vi "故障告警分析.vi"(8 "告警代码":u16, 9 "故障代码":u16, 10 "运行步序":u16, 11 "参数":string) -> (2 "报警内容":T1, 3 "简易报警状态":cluster{"故障状态":string, "报警状态":string}, 5 "platform_alarm_code":string)   [LabVIEW 2016, in "斯坦道CODMn新电路板.lvlib"]
uses:
  Alarm interface/Alarm interface.lvlib
panel:
  # "1、注射泵水样阀口堵塞；\n2、注射泵阀过载或丝杆无动作。"
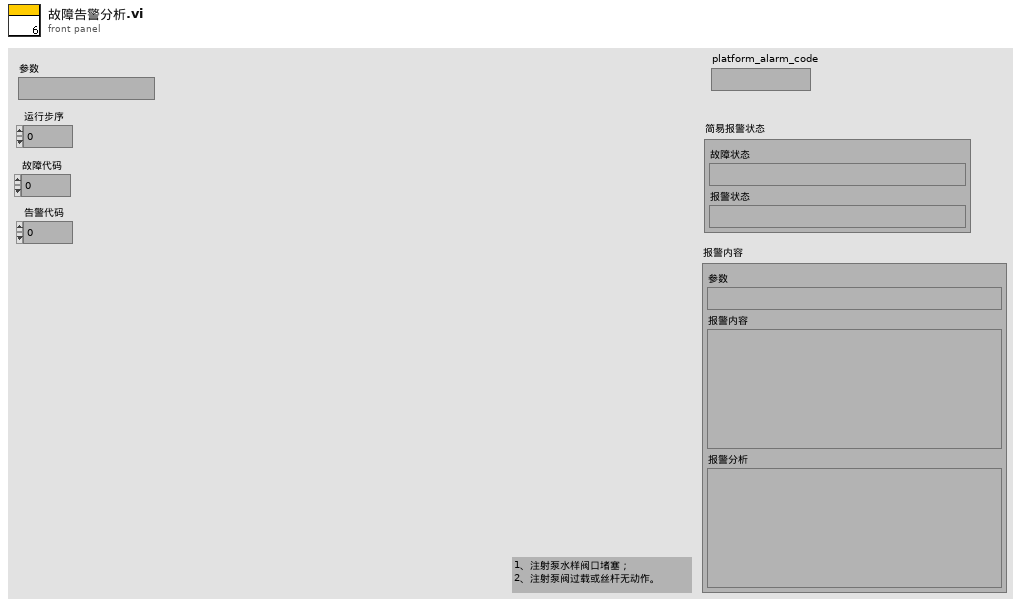
[diagram p1: front panel]
types:
  T1 = cluster{"参数":string, "报警内容":string, "报警分析":string}
  T2 = cluster{"id":string, "code":i32, "level":enum16{"一级", "二级", "三级"}, "message":string, "analysis":string, "platform_alarm_code":string}
  T3 = cluster{"module name":string, "moduleid":i32, "sysid":i32, "content":string, "analysis":string}
  T4 = cluster{"id":string, "ver":string, "type":enum16{"Alarm", "Fault"}, "告警代码":u16}
  T5 = cluster{"id":string, "ver":string, "type":string, "code":u16, "level":enum16{"一级", "二级", "三级"}, "message":string, "analysis":string, "platform_alarm_code":string}
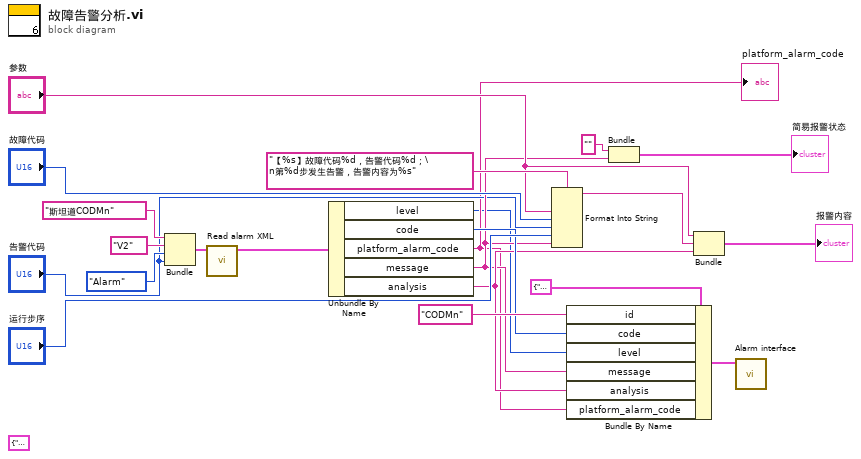
[diagram p0: block diagram]
diagram:
  (unwired) T3 {"module name"="", "moduleid"=0, "sysid"=0, "content"="", "analysis"=""} ("簇")
  n1 = Bundle("id"="斯坦道CODMn", "ver"="V2", "type"=enum16{"Alarm", "Fault"}."Alarm", "告警代码"="告警代码") -> (w5:T4)  [unwired: 1 in]
  n2 = call "Read alarm XML.vi"("筛选输入"=w5) -> ("报警"=w18:T5)  [unwired: 9 in]
  n3 = Unbundle By Name(w18) -> ("level"=w2:enum16{"一级", "二级", "三级"}, "code"=w15:u16, "platform_alarm_code"=w3:string, "message"=w11:string, "analysis"=w13:string)
  "platform_alarm_code" <- w3
  n4 = Format Into String(format string="【%s】故障代码%d，告警代码%d；\n第%d步发生告警，告警内容为%s" ("格式字符串"), "参数", "故障代码", "告警代码", "运行步序", w11) -> (resulting string=w21:string)  [unwired: 2 in, 1 out]
  n5 = Bundle By Name(cluster=T2 {"id"="", "code"=0, "level"=enum."一级", "message"="", "analysis"="", "platform_alarm_code"=""} ("簇"), "id"="CODMn" ("模块名称"), "code"=w15, "level"=w2, "message"=w11, "analysis"=w13, "platform_alarm_code"=w3) -> (w1:T2)
  n6 = Bundle("", "message"=w11) -> (→"简易报警状态":cluster{string, "message":string})  [unwired: 1 in]
  n7 = Bundle("参数"="参数", w21, "analysis"=w13) -> (→"报警内容":cluster{"参数":string, string, "analysis":string})  [unwired: 1 in]
  n8 = call "Alarm interface.vi"("簇"=w1) -> ()  [unwired: 10 in, 1 out]
